vi "Three Motor Mover.vi"() -> ()   [LabVIEW 2017]
panel:
  in  "Low 1":dbl=-100.0 format="%.1f"
  in  "High 1":dbl=100.0 format="%.1f"
  in  "Low 2":dbl=-100.0 format="%.1f"
  in  "High 2":dbl=100.0 format="%.1f"
  in  "Low 3":dbl=-100.0 format="%.1f"
  in  "High 3":dbl=100.0 format="%.1f"
  in  "Zero 3":bool
  in  "Zero 2":bool
  in  "Zero 1":bool
  out "Position 3":dbl format="%.4f"
  in  "Backward Big 3":bool
  in  "Forward Big 3":bool
  in  "Backward Small 3":bool
  in  "Forward Small 3":bool
  in  "Motor 3":refnum<visa-resource-name>="ASRL6::INSTR"
  in  "Large Step Size 3":dbl=10.0 format="%.1f"
  in  "Small Step Size 3":dbl=1.0 format="%_2f"
  out "Position 2":dbl format="%.4f"
  in  "Backward Big 2":bool
  in  "Forward Big 2":bool
  in  "Backward Small 2":bool
  in  "Forward Small 2":bool
  in  "Motor 2":refnum<visa-resource-name>="ASRL5::INSTR"
  in  "Large Step Size 2":dbl=10.0 format="%.1f"
  in  "Small Step Size 2":dbl=1.0 format="%_2f"
  out "Position 1":dbl format="%.4f"
  in  "stop":bool
  in  "Backward Big 1":bool
  in  "Forward Big 1":bool
  in  "Backward Small 1":bool
  in  "Forward Small 1":bool
  in  "Motor 1":refnum<visa-resource-name>="ASRL4::INSTR"
  in  "Large Step Size 1":dbl=10.0 format="%.1f"
  in  "Small Step Size 1":dbl=1.0 format="%_2f"
  # "Limits"
  # "Limits"
  # "Limits"
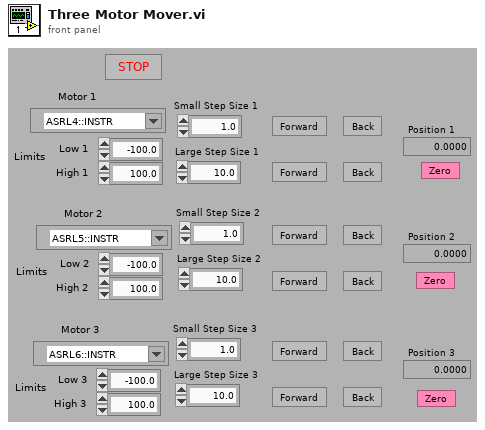
[diagram p1: front panel]
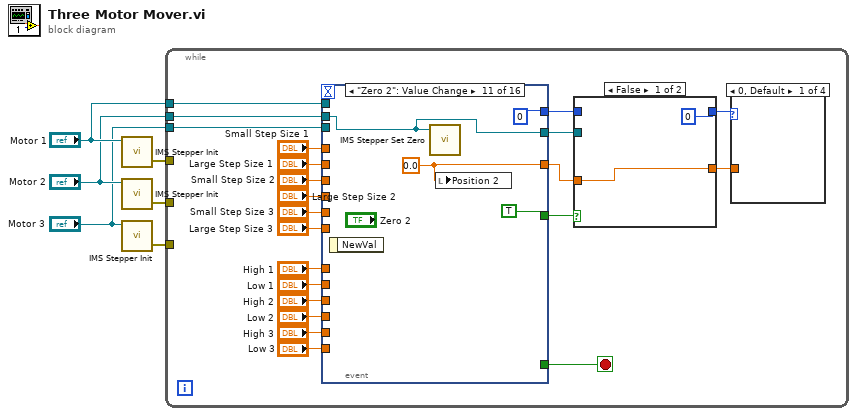
[diagram p0: block diagram]
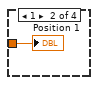
[diagram p2: hidden frame]
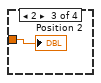
[diagram p3: hidden frame]
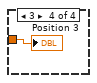
[diagram p4: hidden frame]
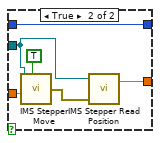
[diagram p5: hidden frame]
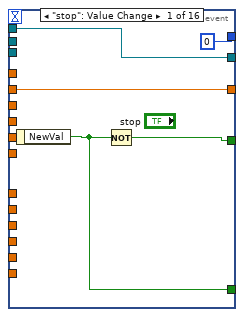
[diagram p6: hidden frame]
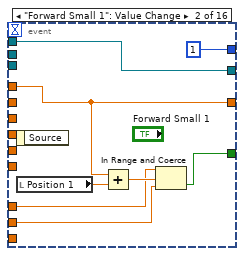
[diagram p7: hidden frame]
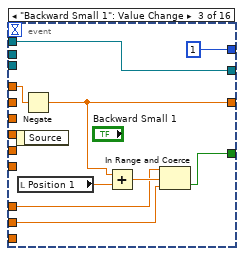
[diagram p8: hidden frame]
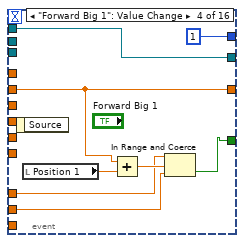
[diagram p9: hidden frame]
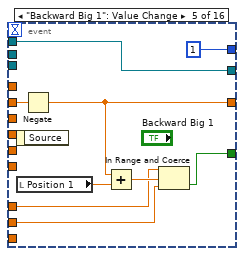
[diagram p10: hidden frame]
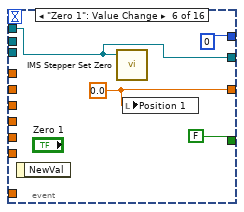
[diagram p11: hidden frame]
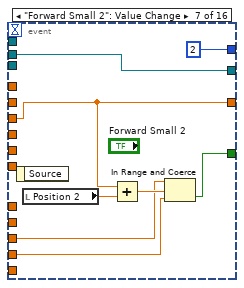
[diagram p12: hidden frame]
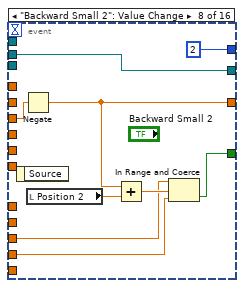
[diagram p13: hidden frame]
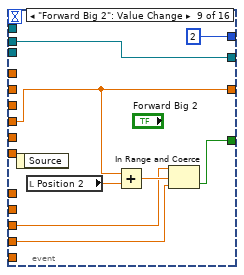
[diagram p14: hidden frame]
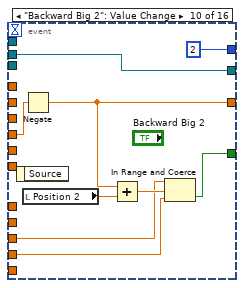
[diagram p15: hidden frame]
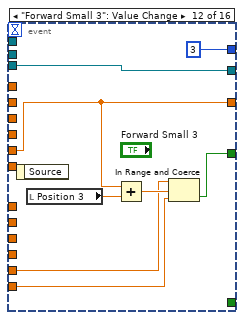
[diagram p16: hidden frame]
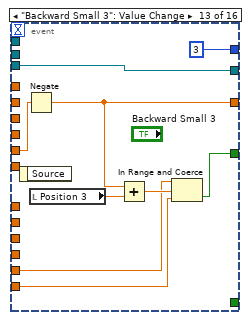
[diagram p17: hidden frame]
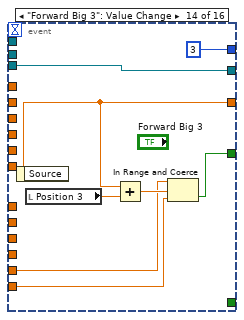
[diagram p18: hidden frame]
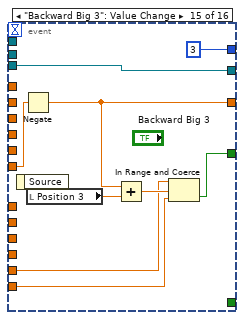
[diagram p19: hidden frame]
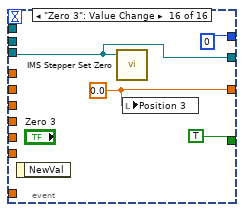
[diagram p20: hidden frame]
diagram:
  n1 = call "IMS Stepper Init.vi"("Instrument Address"="Motor 1") -> ("error out"=w5:errorcluster)  [unwired: 3 in, 1 out]
  n2 = call "IMS Stepper Init.vi"("Instrument Address"="Motor 2") -> ("error out"=w3:errorcluster)  [unwired: 3 in, 1 out]
  n3 = call "IMS Stepper Init.vi"("Instrument Address"="Motor 3") -> ("error out"=w4:errorcluster)  [unwired: 3 in, 1 out]
  n4 = while {
    tunnel: "Motor 1" -> [w21]
    tunnel: w5 -> [_]
    tunnel: w4 -> [_]
    tunnel: w3 -> [_]
    tunnel: "Motor 2" -> [w19]
    tunnel: "Motor 3" -> [w18]
    stop <- w13 stop-if-true
    n5 = event shown="[10] \"Zero 2\": Value Change" {
      selector: _ -> [_ _ _ _ _ _ _ _ _ _ _ _ _ _ _ _]
      dyn-events: _ -> [_ _ _ _ _ _ _ _ _ _ _ _ _ _ _ _]
      timeout: _ -> [_ _ _ _ _ _ _ _ _ _ _ _ _ _ _ _]
      tunnel: w21 -> [w43 w52 w61 w69 w77 w82 _ _ _ _ _ _ _ _ _ _]
      tunnel: "Small Step Size 1" -> [_ w49 w59 _ _ _ _ _ _ _ _ _ _ _ _ _]
      tunnel: "Large Step Size 1" -> [w42 _ _ w62 w78 _ _ _ _ _ _ _ _ _ _ _]
      tunnel: [w43 w52 w61 w69 w77 w82 w89 w98 w106 w114 w117 w127 w135 w144 w152 w155] -> w28
      tunnel: [w42 w49 w55 w62 w72 w79 w85 w93 w102 w110 w118 w124 w132 w141 w148 w156] -> w27
      tunnel: [w41 w45 w56 w63 w73 FALSE ("NewVal") w86 w94 w103 w111 TRUE ("NewVal") w121 w129 w140 w149 TRUE ("NewVal")] -> w20
      tunnel: [0 1 1 1 1 0 2 2 2 2 0 3 3 3 3 0] -> w24
      tunnel: w19 -> [_ _ _ _ _ _ w89 w98 w106 w114 w117 _ _ _ _ _]
      tunnel: w18 -> [_ _ _ _ _ _ _ _ _ _ _ w127 w135 w144 w152 w155]
      tunnel: "Small Step Size 2" -> [_ _ _ _ _ _ w85 w97 _ _ _ _ _ _ _ _]
      tunnel: "Large Step Size 2" -> [_ _ _ _ _ _ _ _ w102 w115 _ _ _ _ _ _]
      tunnel: "Small Step Size 3" -> [_ _ _ _ _ _ _ _ _ _ _ w124 w136 _ _ _]
      tunnel: "Large Step Size 3" -> [_ _ _ _ _ _ _ _ _ _ _ _ _ w141 w153 _]
      tunnel: "High 1" -> [_ w47 w54 w65 w71 _ _ _ _ _ _ _ _ _ _ _]
      tunnel: "Low 1" -> [_ w46 w53 w64 w70 _ _ _ _ _ _ _ _ _ _ _]
      tunnel: "High 2" -> [_ _ _ _ _ _ w84 w92 w101 w109 _ _ _ _ _ _]
      tunnel: "Low 2" -> [_ _ _ _ _ _ w83 w91 w100 w108 _ _ _ _ _ _]
      tunnel: "High 3" -> [_ _ _ _ _ _ _ _ _ _ _ w123 w131 w139 w147 _]
      tunnel: "Low 3" -> [_ _ _ _ _ _ _ _ _ _ _ w122 w130 w138 w146 _]
      tunnel: [w40 _ _ _ _ _ _ _ _ _ _ _ _ _ _ _] -> w13
      event "stop": Value Change {
        n6 = event-data() -> ("NewVal"=w40:bool)  [unwired: 1 in]
        n7 = Not(x=w40) -> (.not. x?=w41:bool)
      }
      event "Forward Small 1": Value Change {
        n8 = event-data() -> ()  [unwired: 1 in, 1 out]
        n9 = local read "Position 1"() -> (w50:dbl)
        n10 = Add(x=w49, y=w50) -> (x+y=w48:dbl)
        n11 = In Range and Coerce(upper limit=w47, x=w48, lower limit=w46) -> (In Range?=w45:bool)  [unwired: 1 out]
      }
      event "Backward Small 1": Value Change {
        n12 = event-data() -> ()  [unwired: 1 in, 1 out]
        n13 = local read "Position 1"() -> (w57:dbl)
        n14 = Negate(x=w59) -> (-x=w55:dbl)
        n15 = Add(x=w55, y=w57) -> (x+y=w58:dbl)
        n16 = In Range and Coerce(upper limit=w54, x=w58, lower limit=w53) -> (In Range?=w56:bool)  [unwired: 1 out]
      }
      event "Forward Big 1": Value Change {
        n17 = event-data() -> ()  [unwired: 1 in, 1 out]
        n18 = local read "Position 1"() -> (w66:dbl)
        n19 = Add(x=w62, y=w66) -> (x+y=w67:dbl)
        n20 = In Range and Coerce(upper limit=w65, x=w67, lower limit=w64) -> (In Range?=w63:bool)  [unwired: 1 out]
      }
      event "Backward Big 1": Value Change {
        n21 = event-data() -> ()  [unwired: 1 in, 1 out]
        n22 = local read "Position 1"() -> (w74:dbl)
        n23 = Negate(x=w78) -> (-x=w72:dbl)
        n24 = Add(x=w72, y=w74) -> (x+y=w75:dbl)
        n25 = In Range and Coerce(upper limit=w71, x=w75, lower limit=w70) -> (In Range?=w73:bool)  [unwired: 1 out]
      }
      event "Zero 1": Value Change {
        w79 = 0.0 ("Large Step Size 3")
        n26 = event-data() -> ()  [unwired: 1 in, 1 out]
        n27 = call "IMS Stepper Set Zero.vi"("Instrument Address"=w82) -> ()  [unwired: 2 in, 1 out]
        n28 = local write "Position 1"(w79) -> ()
      }
      event "Forward Small 2": Value Change {
        n29 = event-data() -> ()  [unwired: 1 in, 1 out]
        n30 = local read "Position 2"() -> (w87:dbl)
        n31 = Add(x=w85, y=w87) -> (x+y=w88:dbl)
        n32 = In Range and Coerce(upper limit=w84, x=w88, lower limit=w83) -> (In Range?=w86:bool)  [unwired: 1 out]
      }
      event "Backward Small 2": Value Change {
        n33 = event-data() -> ()  [unwired: 1 in, 1 out]
        n34 = Negate(x=w97) -> (-x=w93:dbl)
        n35 = local read "Position 2"() -> (w95:dbl)
        n36 = Add(x=w93, y=w95) -> (x+y=w96:dbl)
        n37 = In Range and Coerce(upper limit=w92, x=w96, lower limit=w91) -> (In Range?=w94:bool)  [unwired: 1 out]
      }
      event "Forward Big 2": Value Change {
        n38 = event-data() -> ()  [unwired: 1 in, 1 out]
        n39 = local read "Position 2"() -> (w104:dbl)
        n40 = Add(x=w102, y=w104) -> (x+y=w105:dbl)
        n41 = In Range and Coerce(upper limit=w101, x=w105, lower limit=w100) -> (In Range?=w103:bool)  [unwired: 1 out]
      }
      event "Backward Big 2": Value Change {
        n42 = event-data() -> ()  [unwired: 1 in, 1 out]
        n43 = Negate(x=w115) -> (-x=w110:dbl)
        n44 = local read "Position 2"() -> (w112:dbl)
        n45 = Add(x=w110, y=w112) -> (x+y=w113:dbl)
        n46 = In Range and Coerce(upper limit=w109, x=w113, lower limit=w108) -> (In Range?=w111:bool)  [unwired: 1 out]
      }
      event "Zero 2": Value Change {
        w118 = 0.0 ("Large Step Size 3")
        n47 = event-data() -> ()  [unwired: 1 in, 1 out]
        n48 = call "IMS Stepper Set Zero.vi"("Instrument Address"=w117) -> ()  [unwired: 2 in, 1 out]
        n49 = local write "Position 2"(w118) -> ()
      }
      event "Forward Small 3": Value Change {
        n50 = event-data() -> ()  [unwired: 1 in, 1 out]
        n51 = local read "Position 3"() -> (w125:dbl)
        n52 = Add(x=w124, y=w125) -> (x+y=w126:dbl)
        n53 = In Range and Coerce(upper limit=w123, x=w126, lower limit=w122) -> (In Range?=w121:bool)  [unwired: 1 out]
      }
      event "Backward Small 3": Value Change {
        n54 = event-data() -> ()  [unwired: 1 in, 1 out]
        n55 = Negate(x=w136) -> (-x=w132:dbl)
        n56 = local read "Position 3"() -> (w133:dbl)
        n57 = Add(x=w132, y=w133) -> (x+y=w134:dbl)
        n58 = In Range and Coerce(upper limit=w131, x=w134, lower limit=w130) -> (In Range?=w129:bool)  [unwired: 1 out]
      }
      event "Forward Big 3": Value Change {
        n59 = event-data() -> ()  [unwired: 1 in, 1 out]
        n60 = local read "Position 3"() -> (w142:dbl)
        n61 = Add(x=w141, y=w142) -> (x+y=w143:dbl)
        n62 = In Range and Coerce(upper limit=w139, x=w143, lower limit=w138) -> (In Range?=w140:bool)  [unwired: 1 out]
      }
      event "Backward Big 3": Value Change {
        n63 = event-data() -> ()  [unwired: 1 in, 1 out]
        n64 = Negate(x=w153) -> (-x=w148:dbl)
        n65 = local read "Position 3"() -> (w150:dbl)
        n66 = Add(x=w148, y=w150) -> (x+y=w151:dbl)
        n67 = In Range and Coerce(upper limit=w147, x=w151, lower limit=w146) -> (In Range?=w149:bool)  [unwired: 1 out]
      }
      event "Zero 3": Value Change {
        w156 = 0.0 ("Large Step Size 3")
        n68 = event-data() -> ()  [unwired: 1 in, 1 out]
        n69 = call "IMS Stepper Set Zero.vi"("Instrument Address"=w155) -> ()  [unwired: 2 in, 1 out]
        n70 = local write "Position 3"(w156) -> ()
      }
    }
    n71 = case shown="False" w20 {
      tunnel: w28 -> [_ w37]
      tunnel: w27 -> [w32 w36]
      tunnel: [w32 w35] -> w22
      tunnel: [0 w34] -> w23
      tunnel: w24 -> [_ w34]
      frame False {
      }
      frame True {
        n72 = call "IMS Stepper Move.vi"("Instrument Address"=w37, "Distance"=w36, "Mode"=TRUE) -> ("error out"=w39:errorcluster)  [unwired: 2 in]
        n73 = call "IMS Stepper Read Position.vi"("error in (no error)"=w39, "Instrument Address"=w37) -> ("Response"=w35:dbl)  [unwired: 1 in, 1 out]
      }
    }
    n74 = case shown="0, Default" w23 {
      tunnel: w22 -> [_ w29 w30 w31]
      frame 0, Default {
      }
      frame 1 {
        "Position 1" <- w29
      }
      frame 2 {
        "Position 2" <- w30
      }
      frame 3 {
        "Position 3" <- w31
      }
    }
  }
